vi "Run Tests.vi"(8 "error in":errorcluster, 11 "Report Path in":path) -> (0 "error out":errorcluster, 3 "Report Path Out":path)   [LabVIEW 2020, in "serenial.io-ase.test.lvlib"]
uses:
  serenial.io-ase.test.lvlib
  <vilib>/addons/_JKI Toolkits/Caraya/classes/Test Suite/Define Test Suite (Default).vi
  <vilib>/addons/_JKI Toolkits/Caraya/classes/Test Suite/Test Suite.lvclass
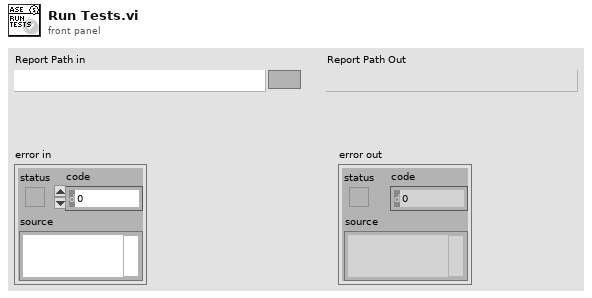
[diagram p1: front panel]
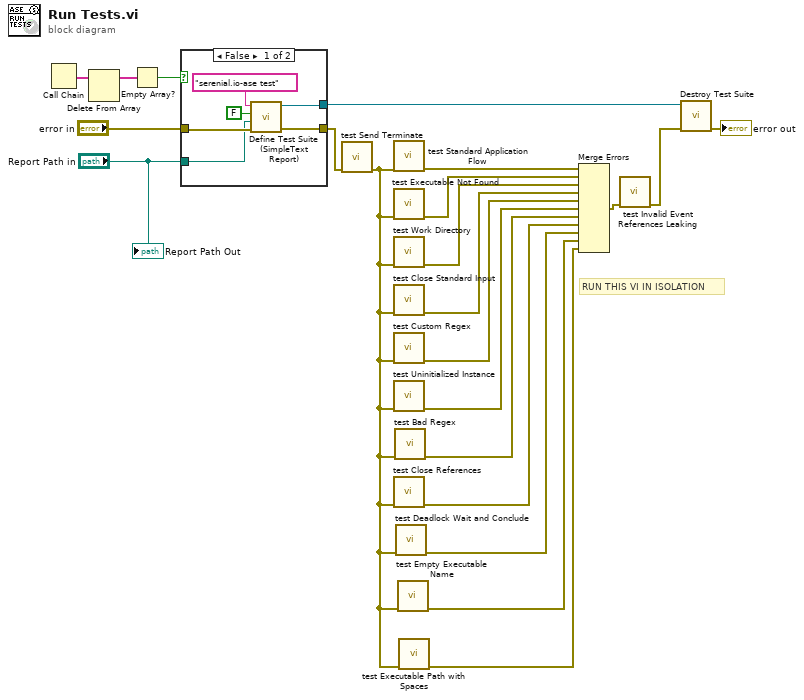
[diagram p0: block diagram]
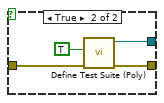
[diagram p2: hidden frame]
diagram:
  # "RUN THIS VI IN ISOLATION"
  n1 = Call Chain() -> (call chain=w13:string[])
  n2 = Delete From Array(array=w13) -> (array with subset deleted=w12:string[])  [unwired: 2 in, 1 out]
  n3 = Empty Array?(array=w12) -> (empty?=w11:bool)
  n4 = case shown="False" w11 {
    tunnel: "error in" -> [w26 w32]
    tunnel: [w28 w31] -> w14
    tunnel: [w27 w30] -> w7
    tunnel: "Report Path in" -> [w25 _]
    frame False {
      n5 = call <vilib>:"Define Test Suite (SimpleText Report).vi"("error in (no error)"=w26, "Report Path"=w25, "Interactive"=FALSE, "Label (VI Title)"="serenial.io-ase test") -> ("error out"=w27:errorcluster, "Test Suite"=w28:refnum<class "Test Suite.lvclass">)  [unwired: 6 in]
    }
    frame True {
      n6 = call-poly <vilib>:"Define Test Suite (Poly).vi"("error in (no error)"=w32, "Interactive"=TRUE) -> ("error out"=w30:errorcluster, "Test Suite"=w31:refnum<class "Test Suite.lvclass">)  [unwired: 8 in]
    }
  }
  n7 = call "test Send Terminate.vi"("error in"=w7) -> ("error out"=w2:errorcluster)  [unwired: 10 in]
  n8 = call "test Standard Application Flow.vi"("error in"=w2) -> ("error out"=w22:errorcluster)  [unwired: 10 in]
  n9 = call "test Executable Not Found.vi"("error in"=w2) -> ("error out"=w21:errorcluster)  [unwired: 10 in]
  n10 = call "test Work Directory.vi"("error in"=w2) -> ("error out"=w20:errorcluster)  [unwired: 10 in]
  n11 = call "test Close Standard Input.vi"("error in"=w2) -> ("error out"=w19:errorcluster)  [unwired: 10 in]
  n12 = call "test Custom Regex.vi"("error in"=w2) -> ("error out"=w18:errorcluster)  [unwired: 10 in]
  n13 = call "test Uninitialized Instance.vi"("error in"=w2) -> ("error out"=w17:errorcluster)  [unwired: 10 in]
  n14 = call "test Close References.vi"("error in"=w2) -> ("error out"=w8:errorcluster)  [unwired: 10 in]
  n15 = call "test Bad Regex.vi"("error in"=w2) -> ("error out"=w9:errorcluster)  [unwired: 10 in]
  n16 = call "test Deadlock Wait and Conclude.vi"("error in"=w2) -> ("error out"=w6:errorcluster)  [unwired: 10 in]
  n17 = call "test Empty Executable Name.vi"("error in"=w2) -> ("error out"=w3:errorcluster)  [unwired: 10 in]
  n18 = call "test Executable Path with Spaces.vi"("error in"=w2) -> ("error out"=w1:errorcluster)  [unwired: 10 in]
  n19 = Merge Errors(w22, w21, w20, w19, w18, w17, w9, w8, w6, w3, w1) -> (w5:errorcluster)
  n20 = call "test Invalid Event References Leaking.vi"("error in"=w5) -> ("error out"=w4:errorcluster)  [unwired: 10 in]
  n21 = call-dynamic "Destroy Test Suite.vi"("error in (no error)"=w4, "Test Suite in"=w14) -> ("error out"=→"error out":errorcluster)  [unwired: 8 in, 1 out]
  "Report Path Out" <- "Report Path in"
